vi "GetMatlabBoundControlByName.vi"(10 "name":string, 11 "ExperimentID":string) -> (0 "Control":refnum<vi>, 1 "found":bool, 3 "Control Binding":T1)   [LabVIEW 2017]
uses:
  Types/ControlValueChangeEventBindingType.ctl
  Types/MatlabBindingDirectionEnum.ctl
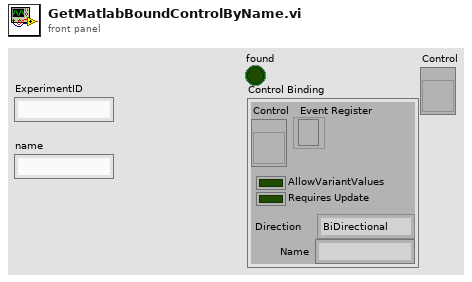
[diagram p1: front panel]
types:
  T1 = typedef "ControlValueChangeEventBindingType.ctl" = cluster{"Control":refnum<vi>, "Event Register":refnum<event-registration>, "AllowVariantValues":bool, "Direction":T2, "Requires Update":bool, "Name":string}
  T2 = typedef "MatlabBindingDirectionEnum.ctl" = enum16{"BiDirectional", "FromMatlab", "ToMatlab"}
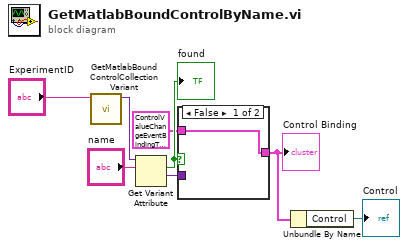
[diagram p0: block diagram]
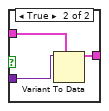
[diagram p2: hidden frame]
diagram:
  n1 = call "GetMatlabBoundControlCollectionVariant.vi"("ExpID"="ExperimentID") -> ("BoundControlCollectionVariant"=w7:variant)  [unwired: 10 in]
  n2 = Get Variant Attribute(Variant=w7, name="name") -> (found=w5:bool, value=w4:variant)  [unwired: 2 in, 2 out]
  "found" <- w5
  n3 = case shown="False" w5 {
    tunnel: w4 -> [_ w12]
    tunnel: T1 {"Control"=refnum, "Event Register"=refnum, "AllowVariantValues"=FALSE, "Direction"=enum."BiDirectional", "Requires Update"=FALSE, "Name"=""} ("Control Binding") -> [w9 w11]
    tunnel: [w9 w10] -> w2
    frame False {
    }
    frame True {
      n4 = Variant To Data(type=w11, Variant=w12) -> (data=w10:T1)  [unwired: 1 in, 1 out]
    }
  }
  "Control Binding" <- w2
  n5 = Unbundle By Name(w2) -> ("Control"=→"Control":refnum<vi>)
